vi "Manual Camera with Grabber.vi"() -> ()   [LabVIEW 2011]
uses:
  Shared Components/GrabberTool Class/GrabberTool Class.lvclass
  Shared Components/Gantry Class/Gantry Class.lvclass
panel:
  out "error out":errorcluster
  in  "Boolean":bool
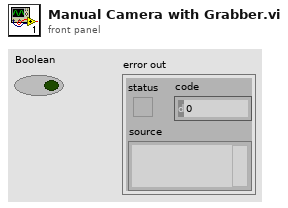
[diagram p1: front panel]
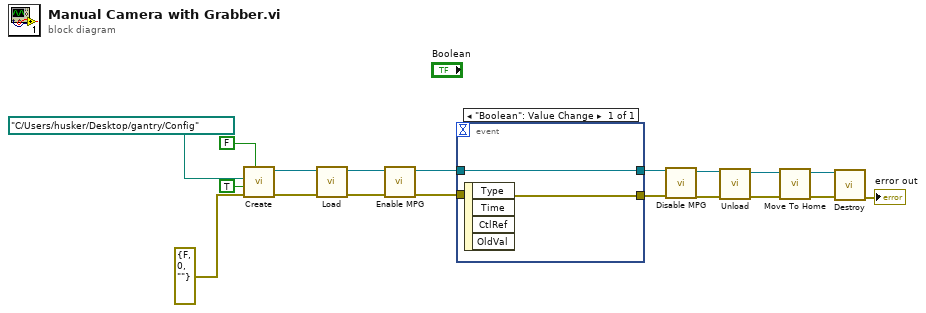
[diagram p0: block diagram]
diagram:
  n1 = call "Create.vi"("Virtual Mode"=FALSE, "error in"=errorcluster {"status"=FALSE, "code"=0, "source"=""}, "HOME?"=TRUE, "Config Folder"=path "C:/Users/husker/Desktop/gantry/Config") -> ("error out"=w16:errorcluster, "Gantry out"=w17:refnum<class "Gantry Class.lvclass">)  [unwired: 6 in]
  n2 = call "Load.vi"("error in"=w16, "Gantry In"=w17) -> ("error out"=w15:errorcluster, "Grabber Tool out"=w18:refnum<class "GrabberTool Class.lvclass">)  [unwired: 8 in]
  n3 = call-dynamic "Enable MPG.vi"("error in"=w15, "Gantry in"=w18) -> ("error out"=w14:errorcluster, "Gantry out"=w19:refnum<class "GrabberTool Class.lvclass">)  [unwired: 8 in]
  n4 = event shown="[0] \"Boolean\": Value Change" {
    selector: _ -> [_]
    dyn-events: _ -> [_]
    timeout: _ -> [_]
    tunnel: w19 -> [w21]
    tunnel: [w21] -> w13
    tunnel: w14 -> [w20]
    tunnel: [w20] -> w10
    event "Boolean": Value Change {
      n5 = event-data() -> ()  [unwired: 1 in, 4 out]
    }
  }
  n6 = call-dynamic "Disable MPG.vi"("error in"=w10, "Gantry in"=w13) -> ("error out"=w11:errorcluster, "Gantry out"=w12:refnum<class "GrabberTool Class.lvclass">)  [unwired: 8 in]
  n7 = call "Unload.vi"("error in"=w11, "GrabberTool in"=w12) -> ("error out"=w2:errorcluster, "Gantry out"=w4:refnum<class "Gantry Class.lvclass">)  [unwired: 8 in]
  n8 = call-dynamic "Move To Home.vi"("error in"=w2, "Gantry in"=w4) -> ("error out"=w1:errorcluster, "Gantry out"=w3:refnum<class "Gantry Class.lvclass">)  [unwired: 8 in]
  n9 = call "Destroy.vi"("error in"=w1, "Gantry Class in"=w3) -> ("error out"=→"error out":errorcluster)  [unwired: 9 in]
